vi "GET_Series.vi"(7 "progress ref":refnum<vi>, 8 "error in (no error)":errorcluster, 10 "series URL":string, 11 "ComicVine_class in":refnum<class "series_class.lvclass">) -> (0 "error out":errorcluster, 3 "ComicVine_class out":refnum<class "series_class.lvclass">)   [LabVIEW 2024, in "series_class.lvclass"]
uses:
  series_class.lvclass
  series_class.lvclass/series_class.ctl
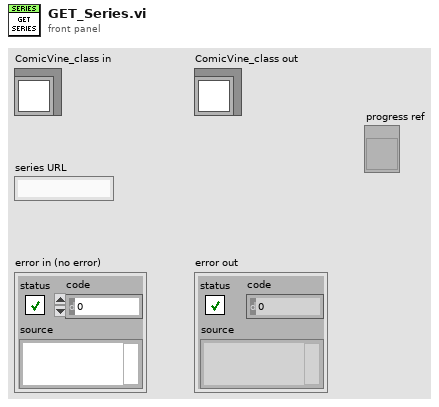
[diagram p1: front panel]
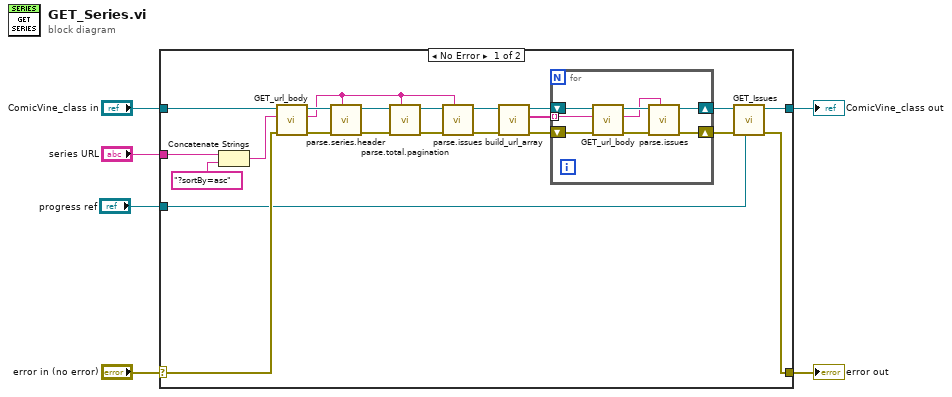
[diagram p0: block diagram]
diagram:
  n1 = case shown="No Error" "error in (no error)" {
    selector: "error in (no error)" -> [w26 w38]
    tunnel: [w9 w38] -> w5
    tunnel: [w11 w37] -> w3
    tunnel: "ComicVine_class in" -> [w28 w37]
    tunnel: "series URL" -> [w21 _]
    tunnel: "progress ref" -> [w7 _]
    frame No Error {
      n2 = Concatenate Strings(w21, "?sortBy=asc") -> (w20:string)
      n3 = call-dynamic "GET_url_body.vi"("error in (no error)"=w26, "url"=w20, "comic_class in"=w28) -> ("error out"=w25:errorcluster, "body"=w13:string, "comic_class out"=w27:refnum<class "series_class.lvclass">)  [unwired: 6 in]
      n4 = call "parse.series.header.vi"("series body"=w13, "error in (no error)"=w25, "ComicVine_class in"=w27) -> ("error out"=w23:errorcluster, "ComicVine_class out"=w24:refnum<class "series_class.lvclass">)  [unwired: 7 in]
      n5 = call "parse.total.pagination.vi"("series body"=w13, "error in (no error)"=w23, "ComicVine_class in"=w24) -> ("error out"=w8:errorcluster, "ComicVine_class out"=w19:refnum<class "series_class.lvclass">)  [unwired: 6 in, 1 out]
      n6 = call "parse.issues.vi"("series body"=w13, "error in (no error)"=w8, "ComicVine_class in"=w19) -> ("error out"=w17:errorcluster, "ComicVine_class out"=w18:refnum<class "series_class.lvclass">)  [unwired: 7 in]
      n7 = call "build_url_array.vi"("error in (no error)"=w17, "ComicVine_class in"=w18) -> ("error out"=w16:errorcluster, "urls"=w14:string[], "ComicVine_class out"=w15:refnum<class "series_class.lvclass">)  [unwired: 7 in]
      n8 = for {
        shift-right: [w30] -> w10
        shift-left: w16 -> [w33]
        shift-right: [w36] -> w12
        shift-left: w15 -> [w32]
        tunnel: w14 -> [w31] mode=indexing
        n9 = call-dynamic "GET_url_body.vi"("error in (no error)"=w33, "url"=w31, "comic_class in"=w32) -> ("error out"=w35:errorcluster, "body"=w29:string, "comic_class out"=w34:refnum<class "series_class.lvclass">)  [unwired: 6 in]
        n10 = call "parse.issues.vi"("series body"=w29, "error in (no error)"=w35, "ComicVine_class in"=w34) -> ("error out"=w30:errorcluster, "ComicVine_class out"=w36:refnum<class "series_class.lvclass">)  [unwired: 7 in]
      }
      n11 = call "GET_Issues.vi"("progress ref"=w7, "error in (no error)"=w10, "series_class in"=w12) -> ("error out"=w9:errorcluster, "series_class out"=w11:refnum<class "series_class.lvclass">)  [unwired: 7 in]
    }
    frame Error {
    }
  }
  "error out" <- w5
  "ComicVine_class out" <- w3
